vi "ROCKET RIGHT.vi"   [LabVIEW 2018]
uses:
  <vilib>/Rock Robotics/WPI/Utilities/WPI_GetSetVariantRefNum.vi
  <vilib>/Rock Robotics/Network Tables/NT Read Number.vi
  Robot Global Data.vi
  <vilib>/Rock Robotics/Network Tables/NT Write Number.vi
types:
  T1 = typedef "WPI_RobotDriveDevRef.ctl" = cluster{"DevStatus":errorcluster, "Motors[]":T2[], "Square Inputs":bool, "Max Output":dbl}
  T2 = typedef "WPI_MotorControlDeviceRef.ctl" = cluster{"DeviceStatus":errorcluster, "Type":T3, "PWM":cluster{"PWM Channel":T4, "DeadBand":T5}, "CAN":cluster{"Device Number":u8, "SetOutput VI Ref":variant, "GetOutput VI Ref":variant, "Enable VI Ref":variant, "Disable VI Ref":variant, "Data":variant}, "Invert":bool, "DIO PWM":cluster{"PWM \"Enable\" Channel":T4, "DIOChannel":T6, "PWM Rate":dbl}}
  T3 = typedef "WPI_MotorControlType.ctl" = enum16{"PWM", "CAN", "DIO PWM"}
  T4 = typedef "FPGA_DIOPWMChannel.ctl" = enum8{"PWM 0", "PWM 1", "PWM 2", "PWM 3", "PWM 4", "PWM 5", "PWM 6", "PWM 7", "PWM 8", "PWM 9", "PWM MXP 0", "PWM MXP 1", "PWM MXP 2", "PWM MXP 3", "PWM MXP 4", "PWM MXP 5", "PWM MXP 6", "PWM MXP 7", "PWM MXP 8", "PWM MXP 9", "Invalid"}
  T5 = typedef "WPI_PWMDeadband.ctl" = cluster{"Name":string, "maxPositivePwm":i32, "minPositivePwm":i32, "centerPwm":i32, "maxNegativePwm":i32, "minNegativePwm":i32, "angularRange":u16}
  T6 = typedef "FPGA_DIOChannel.ctl" = enum8{"DIO 0", "DIO 1", "DIO 2", "DIO 3", "DIO 4", "DIO 5", "DIO 6", "DIO 7", "DIO 8", "DIO 9", "DIO MXP 0", "DIO MXP 1", "DIO MXP 2", "DIO MXP 3", "DIO MXP 4", "DIO MXP 5", "DIO MXP 6", "DIO MXP 7", "DIO MXP 8", "DIO MXP 9", "DIO MXP 10", "DIO MXP 11", "DIO MXP 12", "DIO MXP 13", "DIO MXP 14", "DIO MXP 15", "SPI Port CS1", "SPI Port CS2", "SPI Port CS3", "SPI Port MISO", "SPI Port MOSI", "Invalid"}
  T7 = typedef "WPI_JoystickDevRef.ctl" = cluster{"Device":T8}
  T8 = typedef "WPI_JoystickDeviceEnum.ctl" = enum16{"USB 0", "USB 1", "USB 2", "USB 3", "USB 4", "USB 5"}
  T9 = cluster{"Buttons[0]":bool, "Buttons[1]":bool, "Buttons[2]":bool, "Buttons[3]":bool, "Buttons[4]":bool, "Buttons[5]":bool, "Buttons[6]":bool, "Buttons[7]":bool, "Buttons[8]":bool}
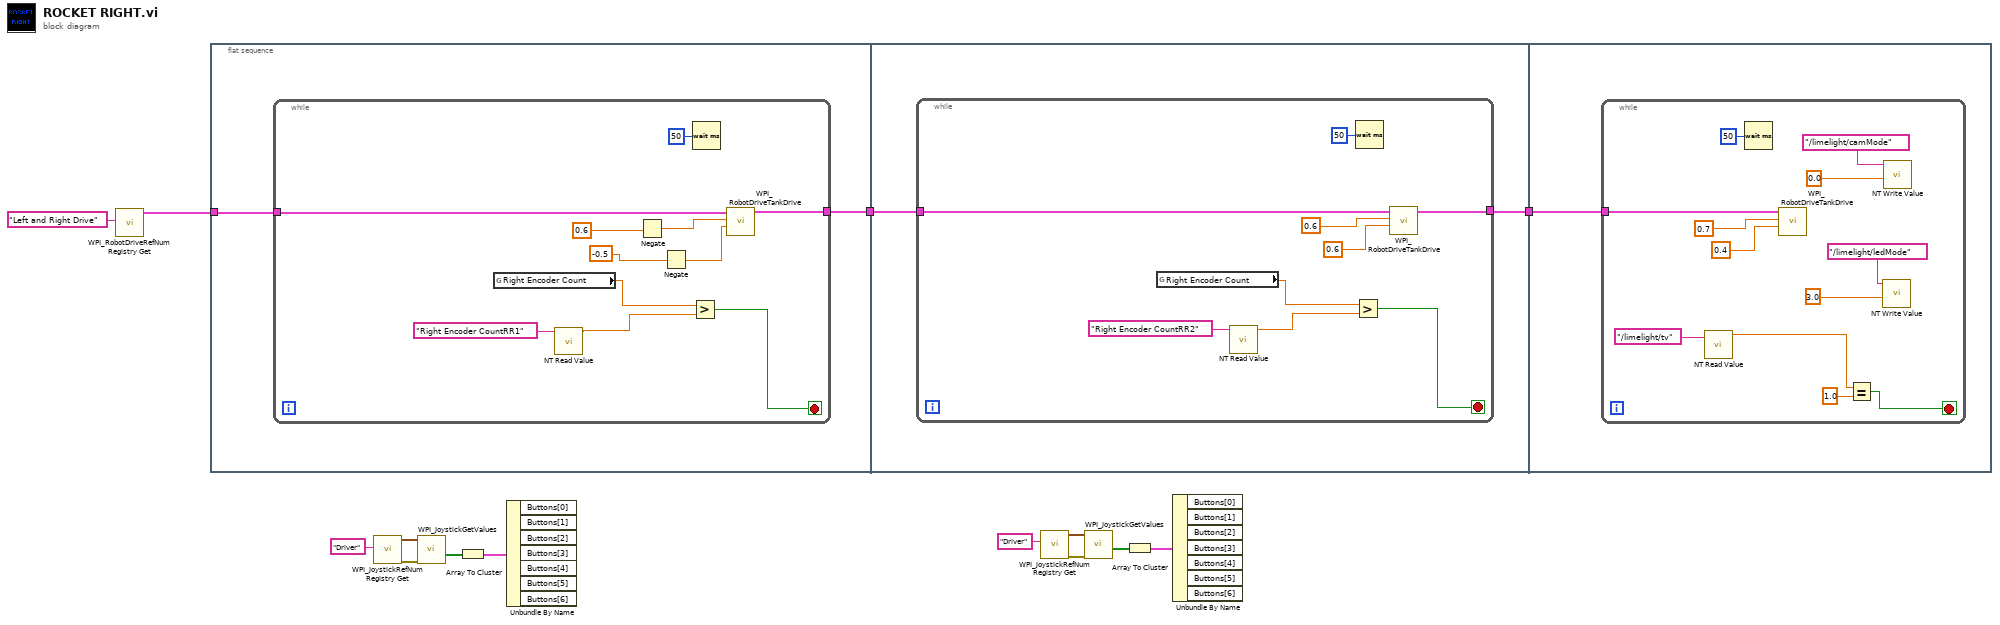
[diagram p0: block diagram]
diagram:
  n1 = call <vilib>:"WPI_RobotDriveRefNum Registry Get.vi"("refnum name"="Left and Right Drive") -> ("RobotDriveDevRef"=w11:T1)  [unwired: 9 in, 1 out]
  n2 = flat-sequence {
    tunnel: w11 -> [w15]
    tunnel: [w16] -> w14
    tunnel: w14 -> [w28]
    tunnel: [w29] -> w13
    tunnel: w13 -> [w39]
    frame #0 {
      n3 = while {
        tunnel: [w26] -> w16
        tunnel: w15 -> [w25]
        stop <- w19 stop-if-true
        n4 = global read "Robot Global Data.vi" "Right Encoder Count"() -> (w24:dbl)
        n5 = call-poly <vilib>:"NT Read Value.vi"("Name"="Right Encoder CountRR1") -> ("Numeric"=w17:dbl)  [unwired: 9 in, 1 out]
        n6 = Negate(x=0.6 ("X axis value")) -> (-x=w22:dbl)
        n7 = Negate(x=-0.5 ("Y axis value")) -> (-x=w20:dbl)
        n8 = Greater?(x=w24, y=w17) -> (0:w19:bool)
        n9 = Wait (ms)(milliseconds to wait=u32 50) -> ()  [unwired: 1 out]
        n10 = call <vilib>:"WPI_RobotDriveTankDrive.vi"("Right axis value"=w20, "Left axis value"=w22, "RobotDriveDevRef"=w25) -> ("RobotDriveDevRef"=w26:T1)  [unwired: 6 in, 2 out]
      }
    }
    frame #1 {
      n11 = while {
        tunnel: [w35] -> w29
        tunnel: w28 -> [w33]
        stop <- w32 stop-if-true
        n12 = global read "Robot Global Data.vi" "Right Encoder Count"() -> (w34:dbl)
        n13 = call-poly <vilib>:"NT Read Value.vi"("Name"="Right Encoder CountRR2") -> ("Numeric"=w30:dbl)  [unwired: 9 in, 1 out]
        n14 = Greater?(x=w34, y=w30) -> (0:w32:bool)
        n15 = Wait (ms)(milliseconds to wait=u32 50) -> ()  [unwired: 1 out]
        n16 = call <vilib>:"WPI_RobotDriveTankDrive.vi"("Right axis value"=0.6 ("Y axis value"), "Left axis value"=0.6 ("X axis value"), "RobotDriveDevRef"=w33) -> ("RobotDriveDevRef"=w35:T1)  [unwired: 6 in, 2 out]
      }
    }
    frame #2 {
      n17 = while {
        tunnel: w39 -> [w50]
        stop <- w41 stop-if-true
        n18 = call-poly <vilib>:"NT Read Value.vi"("Name"="/limelight/tv") -> ("Numeric"=w44:dbl)  [unwired: 9 in, 1 out]
        n19 = Wait (ms)(milliseconds to wait=u32 50) -> ()  [unwired: 1 out]
        n20 = call <vilib>:"WPI_RobotDriveTankDrive.vi"("Right axis value"=0.4 ("Y axis value"), "Left axis value"=0.7 ("X axis value"), "RobotDriveDevRef"=w50) -> ()  [unwired: 6 in, 3 out]
        n21 = Equal?(x=w44, y=1.0) -> (x = y?=w41:bool)
        n22 = call-poly <vilib>:"NT Write Value.vi"("Numeric"=3.0, "Name"="/limelight/ledMode") -> ()  [unwired: 9 in, 1 out]
        n23 = call-poly <vilib>:"NT Write Value.vi"("Numeric"=0.0, "Name"="/limelight/camMode") -> ()  [unwired: 9 in, 1 out]
      }
    }
  }
  n24 = call <vilib>:"WPI_JoystickRefNum Registry Get.vi"("refnum name"="Driver") -> ("error out"=w10:errorcluster, "JoystickDevRef"=w9:T7)  [unwired: 9 in]
  n25 = call <vilib>:"WPI_JoystickGetValues.vi"("error in (no error)"=w10, "JoystickDevRef"=w9) -> ("Buttons"=w8:bool[])  [unwired: 5 in, 4 out]
  n26 = Array To Cluster(array=w8) -> (cluster=w7:T9)
  n27 = Unbundle By Name(w7) -> ()  [unwired: 7 out]
  n28 = call <vilib>:"WPI_JoystickRefNum Registry Get.vi"("refnum name"="Driver") -> ("error out"=w5:errorcluster, "JoystickDevRef"=w4:T7)  [unwired: 9 in]
  n29 = call <vilib>:"WPI_JoystickGetValues.vi"("error in (no error)"=w5, "JoystickDevRef"=w4) -> ("Buttons"=w3:bool[])  [unwired: 5 in, 4 out]
  n30 = Array To Cluster(array=w3) -> (cluster=w2:T9)
  n31 = Unbundle By Name(w2) -> ()  [unwired: 7 out]
